vi "ReturnToNormalMode.vi"(8 "error in (no error)":errorcluster, 11 "Ref":T1) -> (0 "error out":errorcluster, 3 "Ref":T1)   [LabVIEW 2019, in "Diagnostics Host Automation API.lvlib"]
uses:
  Diagnostics Host Automation API.lvlib
  Addon/Addon Shared/Types/HostAutomation.Ref.ctl
  <vilib>/NI/STM/TCP/TCP Connection Info.ctl
  <vilib>/NI/STM/SubVIs/MetaDataElement.ctl
  Addon/Addon Shared/Types/DTC.Codes.ctl
  <vilib>/NI/NI VeriStand Addon Network Comm/Shared/NI VeriStand Addon Network Comm Shared.lvlib
  <vilib>/NI/STM/NI STM.lvlib
  Addon/Addon Shared/Diagnostics Addon Shared.lvlib
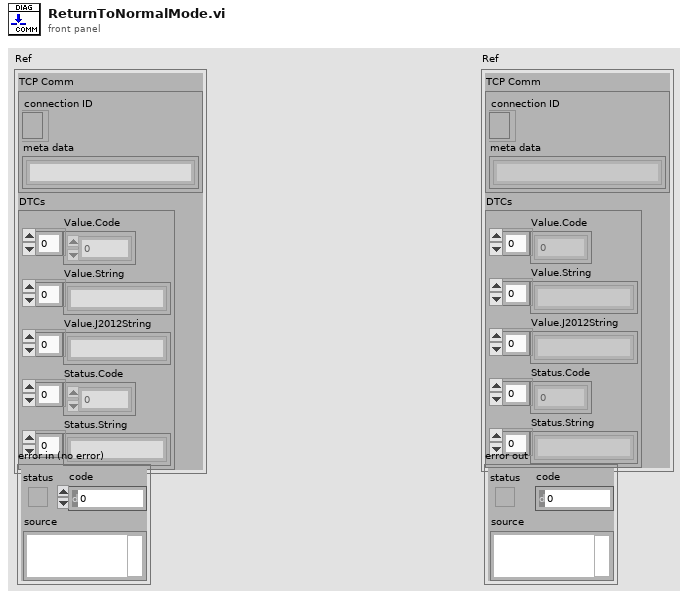
[diagram p1: front panel]
types:
  T1 = typedef "Diagnostics Addon Shared.lvlib/HostAutomation.Ref.ctl" = cluster{"TCP Comm":T2, "DTCs":T4}
  T2 = typedef "NI STM.lvlib/TCP Connection Info.ctl" = cluster{"connection ID":refnum<k5>, "meta data":T3[]}
  T3 = typedef "NI STM.lvlib/MetaDataElement.ctl" = string
  T4 = typedef "Diagnostics Addon Shared.lvlib/DTC.Codes.ctl" = cluster{"Value.Code":dbl[], "Value.String":string[], "Value.J2012String":string[], "Status.Code":dbl[], "Status.String":string[]}
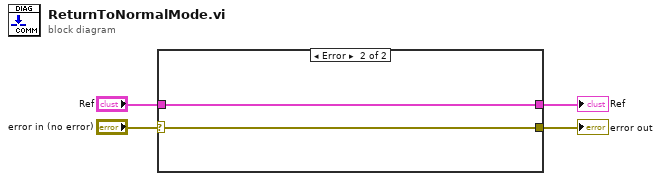
[diagram p0: block diagram]
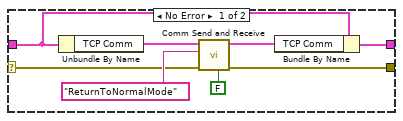
[diagram p2: hidden frame]
diagram:
  n1 = case shown="Error" "error in (no error)" {
    selector: "error in (no error)" -> [w10 w14]
    tunnel: "Ref" -> [w7 w13]
    tunnel: [w5 w13] -> w3
    tunnel: [w12 w14] -> w2
    frame No Error {
      n2 = Unbundle By Name(w7) -> ("TCP Comm"=w8:T2)
      n3 = call <vilib>:"Comm Send and Receive.vi"("Resp Required?"=FALSE, "error in (no error)"=w10, "Name"="ReturnToNormalMode", "connection info"=w8) -> ("error out"=w12:errorcluster, "connection info"=w6:T2)  [unwired: 4 in, 2 out]
      n4 = Bundle By Name(cluster=w7, "TCP Comm"=w6) -> (w5:T1)
    }
    frame Error {
    }
  }
  "Ref" <- w3
  "error out" <- w2
